vi "PWM_v1.vi"(8 "error in":errorcluster, 11 "PWM Sel.":enum16{"1", "2", "3", "4", "5", "6"}(ring)) -> (0 "error out":errorcluster={"status"=FALSE, "code"=200040, "source"="Property Node (arg 1) in PWM_v1.vi"}, 3 "Amp Gain":dbl[](array[numeric])=[2.051898140791966])   [LabVIEW 2021]
uses:
  <vilib>/DAQmx/write.llb/DAQmx Write (Analog 1D Wfm NChan NSamp).vi
  <vilib>/DAQmx/read.llb/DAQmx Read (Analog 1D Wfm NChan NSamp).vi
  <vilib>/DAQmx/create/channels.llb/DAQmx Create Channel (AO-Voltage-Basic).vi
  <vilib>/DAQmx/create/channels.llb/DAQmx Create Channel (AI-Voltage-Basic).vi
  <vilib>/DAQmx/configure/timing.llb/DAQmx Timing (Sample Clock).vi
  <vilib>/measure/madcrms.llb/Basic Averaged DC-RMS for N Chan.vi
  <vilib>/measure/mascope.llb/Amplitude and Levels N chan.vi
  <vilib>/DAQmx/miscellaneous.llb/DAQmx Fill In Error Info.vi
  <resource>/objmgr/daqmx.rc
  <vilib>/measure/NI_MABase.lvlib
  <vilib>/measure/NI_MAPro.lvlib
panel:
  out "RMS Gain":dbl[](array[numeric])=[2.2147861826574564]
  out "DC In":dbl[](array[numeric])=[5.0] format="%.2p"
  out "RMS In":dbl[](array[numeric])=[7.0710678118654755] format="%.2p"
  out "RMS Out":dbl[](array[numeric])=[3.1926638640038427] format="%.2p"
  in  "Sample Rate AI":dbl=50000.0
  in  "Sample Rate AO":dbl=50000.0
  in  "Sample Clock Source AI":tag="OnboardClock"
  in  "Sample Mode AI":i32(ring)=10178 items=["Finite Samples"=10178, "Continuous Samples"=10123, "Hardware Timed Single Point"=12522]
  in  "Number of Samples AI":i32=500
  out "DC Out":dbl[](array[numeric])=[2.0936977209503738] format="%.2p"
  out "Amplitude Out":dbl[](array[numeric])=[4.854499013364962] format="%.2p"
  out "High Out":dbl[](array[numeric])=[4.863375920862381] format="%.2p"
  out "Low Out":dbl[](array[numeric])=[0.008876907497418828] format="%.2p"
  out "Amplitude In":dbl[](array[numeric])=[9.9609375] format="%.2p"
  out "Low In":dbl[](array[numeric])=[0.01953125] format="%.2p"
  out "High In":dbl[](array[numeric])=[9.98046875] format="%.2p"
  in  "Sample Mode AO":i32(ring)=10123 items=["Finite Samples"=10178, "Continuous Samples"=10123, "Hardware Timed Single Point"=12522]
  out "Output Waveform":waveform(dbl)[](graph)=[{"t0"=timestamp(3719340435.858088 s since 1904-01-01), "dt"=1.9999999999999998e-05, "Y"=array[500 elements], "attributes"=variant("NI_ChannelName"=variant(string "BONTS_Mod1/ai24"), "NI_UnitDescription"=variant(string "Volts"))}]
  out "Input Waveform":waveform(dbl)[](graph)=[{"t0"=timestamp(0 s since 1904-01-01), "dt"=2e-05, "Y"=[10.0, 10.0, 10.0, 10.0, 10.0, 10.0, 10.0, 10.0, 0.0, 0.0, 0.0, 0.0, 0.0, 0.0, 0.0, 10.0, 10.0, 10.0, 10.0, 10.0, 10.0, 10.0, 0.0, 0.0, 0.0, 0.0, 0.0, 0.0, 0.0, 10.0, 10.0, 10.0, 10.0, 10.0, 10.0, 10.0, 0.0, 0.0, 0.0, 0.0, 0.0, 0.0, 0.0, 10.0, 10.0, 10.0, 10.0, 10.0, 10.0, 10.0, 0.0, 0.0, 0.0, 0.0, 0.0, 0.0, 0.0, 0.0, 10.0, 10.0, 10.0, 10.0, 10.0, 10.0, 10.0, 0.0, 0.0, 0.0, 0.0, 0.0, 0.0, 0.0, 10.0, 10.0, 10.0, 10.0, 10.0, 10.0, 10.0, 0.0, 0.0, 0.0, 0.0, 0.0, 0.0, 0.0, 10.0, 10.0, 10.0, 10.0, 10.0, 10.0, 10.0, 0.0, 0.0, 0.0, 0.0, 0.0, 0.0, 0.0, 10.0, 10.0, 10.0, 10.0, 10.0, 10.0, 10.0, 10.0, 0.0, 0.0, 0.0, 0.0, 0.0, 0.0, 0.0, 10.0, 10.0, 10.0, 10.0, 10.0, 10.0, 10.0, 0.0, 0.0, 0.0, 0.0, 0.0, 0.0, 0.0, 10.0, 10.0, 10.0, 10.0, 10.0, 10.0, 10.0, 0.0, 0.0, 0.0, 0.0, 0.0, 0.0, 0.0, 10.0, 10.0, 10.0, 10.0, 10.0, 10.0, 10.0, 0.0, 0.0, 0.0, 0.0, 0.0, 0.0, 0.0, 0.0, 10.0, 10.0, 10.0, 10.0, 10.0, 10.0, 10.0, 0.0, 0.0, 0.0, 0.0, 0.0, 0.0, 0.0, 10.0, 10.0, 10.0, 10.0, 10.0, 10.0, 10.0, 0.0, 0.0, 0.0, 0.0, 0.0, 0.0, 0.0, 10.0, 10.0, 10.0, 10.0, 10.0, 10.0, 10.0, 0.0, 0.0, 0.0, 0.0, 0.0, 0.0, 0.0, 10.0, 10.0, 10.0, 10.0, 10.0, 10.0, 10.0, 10.0, 0.0, 0.0, 0.0, 0.0, 0.0, 0.0, 0.0, 10.0, 10.0, 10.0, 10.0, 10.0, 10.0, 10.0, 0.0, 0.0, 0.0, 0.0, 0.0, 0.0, 0.0, 10.0, 10.0, 10.0, 10.0, 10.0, 10.0, 10.0, 0.0, 0.0, 0.0, 0.0, 0.0, 0.0, 0.0, 10.0, 10.0, 10.0, 10.0, 10.0, 10.0, 10.0, 0.0, 0.0, 0.0, 0.0, 0.0, 0.0, 0.0, 0.0, 10.0, 10.0, 10.0, 10.0, 10.0, 10.0, 10.0, 0.0, 0.0, 0.0, 0.0, 0.0, 0.0, 0.0, 10.0, 10.0, 10.0, 10.0, 10.0, 10.0, 10.0, 0.0, 0.0, 0.0, 0.0, 0.0, 0.0, 0.0, 10.0, 10.0, 10.0, 10.0, 10.0, 10.0, 10.0, 0.0, 0.0, 0.0, 0.0, 0.0, 0.0, 0.0, 10.0, 10.0, 10.0, 10.0, 10.0, 10.0, 10.0, 10.0, 0.0, 0.0, 0.0, 0.0, 0.0, 0.0, 0.0, 10.0, 10.0, 10.0, 10.0, 10.0, 10.0, 10.0, 0.0, 0.0, 0.0, 0.0, 0.0, 0.0, 0.0, 10.0, 10.0, 10.0, 10.0, 10.0, 10.0, 10.0, 0.0, 0.0, 0.0, 0.0, 0.0, 0.0, 0.0, 10.0, 10.0, 10.0, 10.0, 10.0, 10.0, 10.0, 0.0, 0.0, 0.0, 0.0, 0.0, 0.0, 0.0, 0.0, 10.0, 10.0, 10.0, 10.0, 10.0, 10.0, 10.0, 0.0, 0.0, 0.0, 0.0, 0.0, 0.0, 0.0, 10.0, 10.0, 10.0, 10.0, 10.0, 10.0, 10.0, 0.0, 0.0, 0.0, 0.0, 0.0, 0.0, 0.0, 10.0, 10.0, 10.0, 10.0, 10.0, 10.0, 10.0, 0.0, 0.0, 0.0, 0.0, 0.0, 0.0, 0.0, 10.0, 10.0, 10.0, 10.0, 10.0, 10.0, 10.0, 10.0, 0.0, 0.0, 0.0, 0.0, 0.0, 0.0, 0.0, 10.0, 10.0, 10.0, 10.0, 10.0, 10.0, 10.0, 0.0, 0.0, 0.0, 0.0, 0.0, 0.0, 0.0, 10.0, 10.0, 10.0, 10.0, 10.0, 10.0, 10.0, 0.0, 0.0, 0.0, 0.0, 0.0, 0.0, 0.0, 10.0, 10.0, 10.0, 10.0, 10.0, 10.0, 10.0, 0.0, 0.0, 0.0, 0.0, 0.0, 0.0, 0.0, 0.0, 10.0, 10.0, 10.0, 10.0, 10.0, 10.0, 10.0, 0.0, 0.0, 0.0, 0.0, 0.0, 0.0, 0.0, 10.0, 10.0, 10.0, 10.0, 10.0, 10.0, 10.0, 0.0, 0.0, 0.0, 0.0, 0.0, 0.0, 0.0, 10.0, 10.0, 10.0, 10.0, 10.0, 10.0, 10.0, 0.0, 0.0, 0.0, 0.0, 0.0, 0.0, 0.0]}]
  in  "Number of Samples AO":i32=500
  in  "Sample Clock Source AO":tag="OnboardClock"
  out "Actual Sample Rate":dbl=50000.0 format="%0.2f"
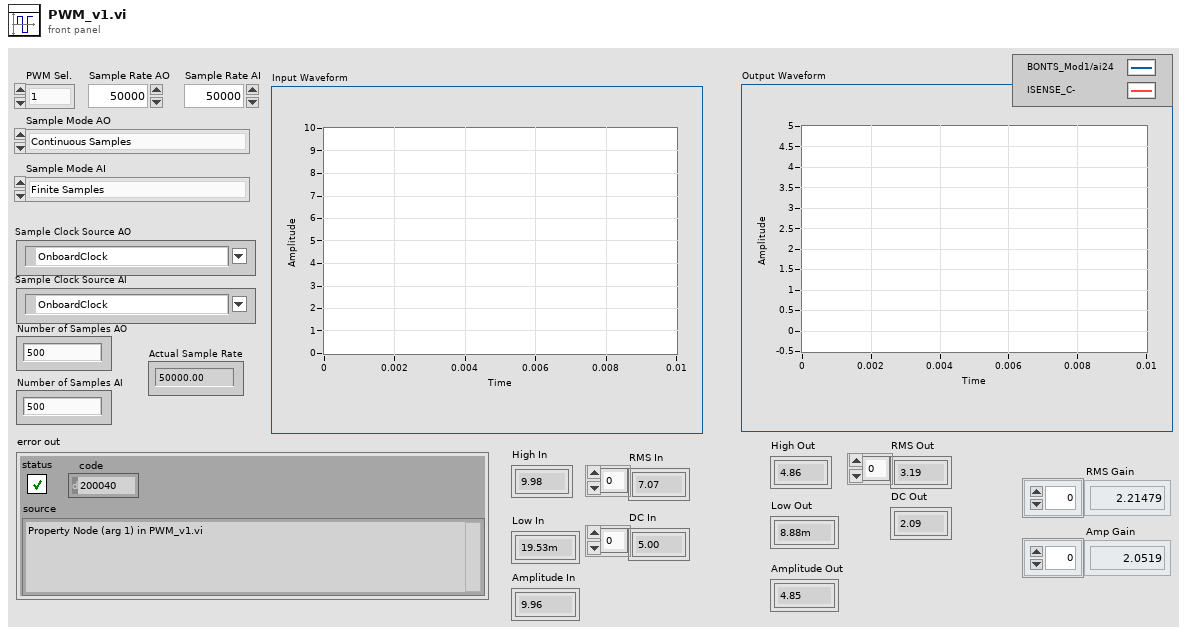
[diagram p1: front panel]
types:
  T1 = cluster{"Waveform Type":u16, "Amplitude":dbl, "Frequency":dbl}[]
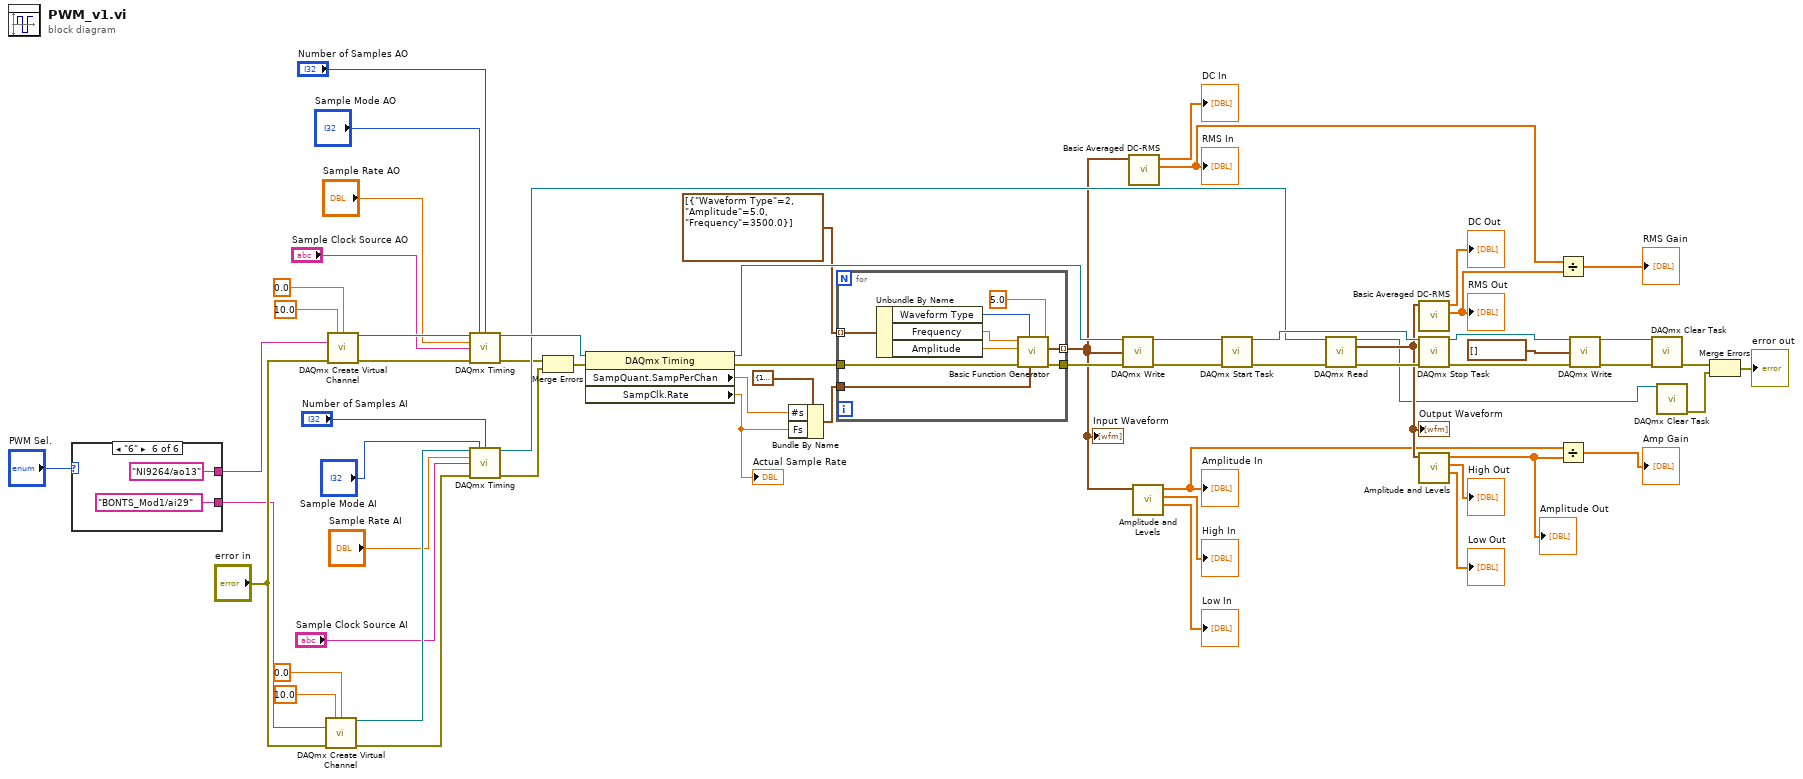
[diagram p0: block diagram]
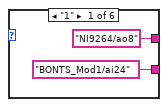
[diagram p2: hidden frame]
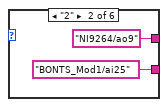
[diagram p3: hidden frame]
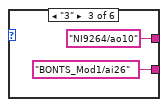
[diagram p4: hidden frame]
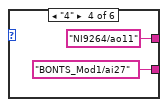
[diagram p5: hidden frame]
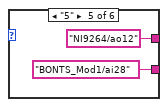
[diagram p6: hidden frame]
diagram:
  n1 = case shown="\"6\"" "PWM Sel." {
    tunnel: ["BONTS_Mod1/ai24" ("Read Channel") "BONTS_Mod1/ai25" ("Read Channel") "BONTS_Mod1/ai26" ("Read Channel") "BONTS_Mod1/ai27" ("Read Channel") "BONTS_Mod1/ai28" ("Read Channel") "BONTS_Mod1/ai29" ("Read Channel")] -> w14
    tunnel: ["NI9264/ao8" ("Write Channel") "NI9264/ao9" ("Write Channel") "NI9264/ao10" ("Write Channel") "NI9264/ao11" ("Write Channel") "NI9264/ao12" ("Write Channel") "NI9264/ao13" ("Write Channel")] -> w37
    frame "1" {
    }
    frame "2" {
    }
    frame "3" {
    }
    frame "4" {
    }
    frame "5" {
    }
    frame "6" {
    }
  }
  n2 = call-poly <vilib>:"DAQmx Create Virtual Channel.vi"("maximum value"=10.0, "minimum value"=0.0, "physical channels"=w14, "error in"="error in") -> ("task out"=w24:refnum<k21>, "error out"=w19:errorcluster)  [unwired: 10 in]
  n3 = call-poly <vilib>:"DAQmx Create Virtual Channel.vi"("maximum value"=10.0, "minimum value"=0.0, "physical channels"=w37, "error in"="error in") -> ("task out"=w59:refnum<k21>, "error out"=w60:errorcluster)  [unwired: 10 in]
  n4 = call-poly <vilib>:"DAQmx Timing.vi"("task/channels in"=w59, "sample mode"="Sample Mode AO", "samples per channel"="Number of Samples AO", "rate"="Sample Rate AO", "source"="Sample Clock Source AO", "error in"=w60) -> ("task out"=w38:refnum<k21>, "error out"=w17:errorcluster)  [unwired: 8 in]
  n5 = call-poly <vilib>:"DAQmx Timing.vi"("task/channels in"=w24, "sample mode"="Sample Mode AI", "samples per channel"="Number of Samples AI", "rate"="Sample Rate AI", "source"="Sample Clock Source AI", "error in"=w19) -> ("task out"=w25:refnum<k21>, "error out"=w16:errorcluster)  [unwired: 8 in]
  n6 = Merge Errors(w17, w16) -> (w18:errorcluster)
  n7 = property class="DAQmx Timing"(reference=w38, error in=w18) -> (reference out=w36:refnum<k21>, error out=w48:errorcluster, "SampQuant.SampPerChan"=w51:dbl, "SampClk.Rate"=w50:dbl)
  "Actual Sample Rate" <- w50
  n8 = Bundle By Name(cluster=cluster{"Fs":dbl, "#s":dbl} {"Fs"=1000.0, "#s"=1000.0} ("sampling info"), "#s"=w51, "Fs"=w50) -> (w56:cluster{"Fs":dbl, "#s":dbl})
  n9 = for {
    tunnel: w48 -> [w82]
    tunnel: w56 -> [w81]
    tunnel: [w80] -> w53
    tunnel: T1 [{"Waveform Type"=2, "Amplitude"=5.0, "Frequency"=3500.0}] ("Output Array") -> [w79] mode=indexing
    tunnel: [w75] -> w9 mode=indexing
    n10 = Unbundle By Name(w79) -> ("Waveform Type"=w78:u16, "Frequency"=w77:dbl, "Amplitude"=w76:dbl)
    n11 = call <vilib>:"Basic Function Generator.vi"("offset"=5.0, "sampling info"=w81, "signal type"=w78, "error in (no error)"=w82, "amplitude"=w76, "frequency"=w77) -> ("error out"=w80:errorcluster, "signal out"=w75:waveform(dbl))  [unwired: 3 in, 1 out]
  }
  "Input Waveform" <- w9
  n12 = call-poly <vilib>:"DAQmx Write.vi"("task/channels in"=w36, "data"=w9, "error in"=w53) -> ("task out"=w55:refnum<k21>, "error out"=w54:errorcluster)  [unwired: 10 in, 1 out]
  n13 = call-poly <vilib>:"Basic Averaged DC-RMS.vi"("signals in"=w9) -> ("RMS values"=w5:dbl[], "DC values"=→"DC In":dbl[])  [unwired: 7 in, 2 out]
  "RMS In" <- w5
  n14 = call-poly <vilib>:"Amplitude and Levels.vi"("signal(s) in"=w9) -> ("low state level"=→"Low In":dbl[], "high state level"=→"High In":dbl[], "amplitude"=w3:dbl[])  [unwired: 7 in, 1 out]
  "Amplitude In" <- w3
  n15 = call <vilib>:"DAQmx Start Task.vi"("task/channels in"=w55, "error in"=w54) -> ("task out"=w49:refnum<k21>, "error out"=w47:errorcluster)  [unwired: 12 in]
  n16 = call-poly <vilib>:"DAQmx Read.vi"("task/channels in"=w25, "error in"=w47) -> ("task out"=w10:refnum<k21>, "data"=w39:waveform(dbl)[], "error out"=w46:errorcluster)  [unwired: 11 in]
  "Output Waveform" <- w39
  n17 = call-poly <vilib>:"Basic Averaged DC-RMS.vi"("signals in"=w39) -> ("RMS values"=w6:dbl[], "DC values"=→"DC Out":dbl[])  [unwired: 7 in, 2 out]
  "RMS Out" <- w6
  n18 = call <vilib>:"DAQmx Stop Task.vi"("task/channels in"=w49, "error in"=w46) -> ("task out"=w33:refnum<k21>, "error out"=w35:errorcluster)  [unwired: 12 in]
  n19 = call-poly <vilib>:"Amplitude and Levels.vi"("signal(s) in"=w39) -> ("low state level"=→"Low Out":dbl[], "high state level"=→"High Out":dbl[], "amplitude"=w2:dbl[])  [unwired: 7 in, 1 out]
  "Amplitude Out" <- w2
  n20 = Divide(x=w5, y=w6) -> (x/y=→"RMS Gain":dbl[])
  n21 = Divide(x=w3, y=w2) -> (x/y=→"Amp Gain":dbl[])
  n22 = call-poly <vilib>:"DAQmx Write.vi"("task/channels in"=w33, "data"=waveform(dbl)[] [], "error in"=w35) -> ("task out"=w32:refnum<k21>, "error out"=w34:errorcluster)  [unwired: 10 in, 1 out]
  n23 = call <vilib>:"DAQmx Clear Task.vi"("task in"=w32, "error in"=w34) -> ("error out"=w12:errorcluster)  [unwired: 13 in]
  n24 = call <vilib>:"DAQmx Clear Task.vi"("task in"=w10) -> ("error out"=w11:errorcluster)  [unwired: 14 in]
  n25 = Merge Errors(w12, w11) -> (→"error out":errorcluster)
